vi "RasterScan.vi"() -> ()   [LabVIEW 2009]
panel:
  in  "Tab Control":T1(tab)=enum."IKI1 + NICMOS"
  in  "Aero-Me: Size":i32=5
  in  "Aero-Me: Step":dbl=50.0
  in  "Iki1: Size":i32=5
  in  "Iki1: Step":dbl=0.1
  in  "Iki2: Size":i32=5
  in  "Iki2: Step":dbl=0.1
  in  "Schnee-Me: Step":dbl=50.0
  in  "Schnee-Me: Size":i32=5
  out "Final Y":dbl
  out "Final X":dbl
  out "Start Y":dbl=53210.0
  out "Start X":dbl=24018.0
  out "Raster Scan":dbl[][](graph)
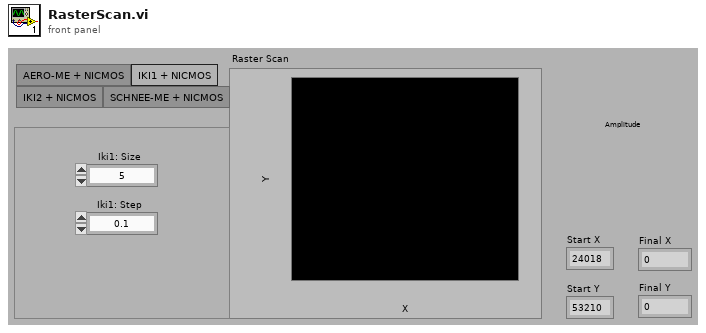
[diagram p1: front panel]
types:
  T1 = enum32{"AERO-ME + NICMOS", "IKI1 + NICMOS", "IKI2 + NICMOS", "SCHNEE-ME + NICMOS"}
  T2 = enum16{"Acquire", "GetAbsolutePosition", "AbsoluteMove", "Release"}
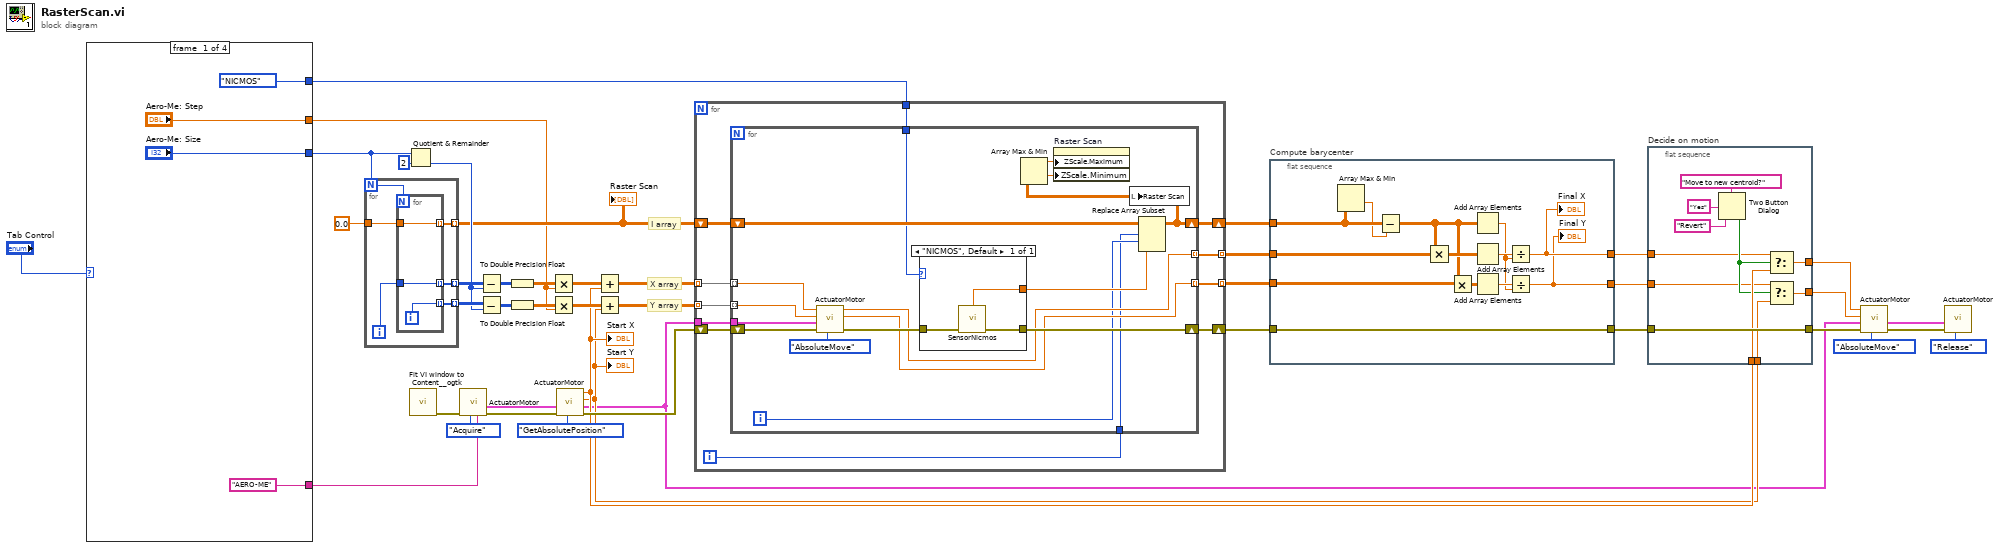
[diagram p0: block diagram]
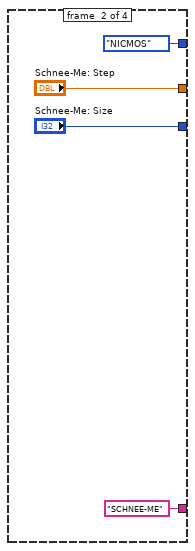
[diagram p2: hidden frame]
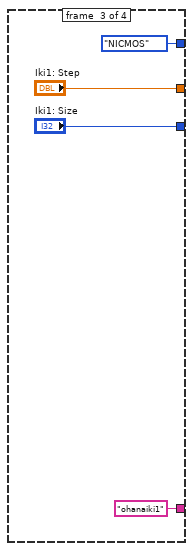
[diagram p3: hidden frame]
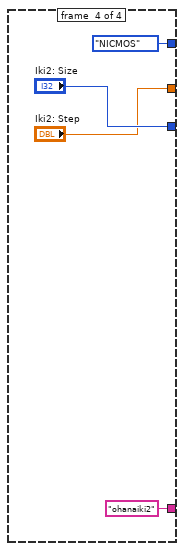
[diagram p4: hidden frame]
diagram:
  # "I array"
  # "Y array"
  # "X array"
  n1 = case shown="\"IKI2 + NICMOS\"" "Tab Control" {
    tunnel: ["Aero-Me: Size" "Schnee-Me: Size" "Iki1: Size" "Iki2: Size"] -> w40
    tunnel: ["Aero-Me: Step" "Schnee-Me: Step" "Iki1: Step" "Iki2: Step"] -> w7
    tunnel: [enum16{"NICMOS"}."NICMOS" ("Sensor") enum16{"NICMOS"}."NICMOS" ("Sensor") enum16{"NICMOS"}."NICMOS" ("Sensor") enum16{"NICMOS"}."NICMOS" ("Sensor")] -> w6
    tunnel: ["AERO-ME" ("Ring Text.Text") "SCHNEE-ME" ("Ring Text.Text") "ohanaiki1" ("Ring Text.Text") "ohanaiki2" ("Ring Text.Text")] -> w5
    frame #0 {
    }
    frame #1 {
    }
    frame #2 {
    }
    frame #3 {
    }
  }
  n2 = for {
    N: w40 -> [w61]
    tunnel: [w64] -> w42 mode=indexing
    tunnel: [w62] -> w41 mode=indexing
    tunnel: 0.0 ("element") -> [w60]
    tunnel: [w59] -> w12 mode=indexing
    i -> [w63]
    n3 = for {
      N: w61 -> [_]
      tunnel: [w67] -> w64 mode=indexing
      tunnel: w63 -> [w67]
      tunnel: [w66] -> w62 mode=indexing
      tunnel: w60 -> [w65]
      tunnel: [w65] -> w59 mode=indexing
      i -> [w66]
    }
  }
  "Raster Scan" <- w12
  n4 = Quotient & Remainder(x=w40, y=2) -> (floor(x/y)=w38:i32)  [unwired: 1 out]
  n5 = call <userlib>:"Fit VI window to Content__ogtk.vi"() -> ("error out"=w4:errorcluster)  [unwired: 6 in, 1 out]
  n6 = call "ActuatorMotor.vi"("Actuator Name"=w5, "Command"=T2."Acquire", "error in (no error)"=w4) -> ("error out"=w27:errorcluster, "RefNum out"=w3:cluster{string, "Variant":variant})  [unwired: 3 in, 2 out]
  n7 = Subtract(x=w42, y=w38) -> (x-y=w36:i32[][])
  n8 = Subtract(x=w41, y=w38) -> (x-y=w33:i32[][])
  n9 = To Double Precision Float(number=w36) -> (double precision float=w35:dbl[][])
  n10 = To Double Precision Float(number=w33) -> (double precision float=w34:dbl[][])
  n11 = Multiply(x=w35, y=w7) -> (x*y=w25:dbl[][])
  n12 = Multiply(x=w34, y=w7) -> (x*y=w23:dbl[][])
  n13 = call "ActuatorMotor.vi"("Command"=T2."GetAbsolutePosition", "error in (no error)"=w27, "RefNum"=w3) -> ("error out"=w31:errorcluster, "RefNum out"=w1:cluster{string, "Variant":variant}, "Y out"=w15:dbl, "X out"=w16:dbl)  [unwired: 3 in]
  "Start X" <- w16
  "Start Y" <- w15
  n14 = Add(x=w25, y=w16) -> (x+y=w24:dbl[][])
  n15 = Add(x=w23, y=w15) -> (x+y=w22:dbl[][])
  n16 = for {
    tunnel: w24 -> [w78] mode=indexing
    tunnel: w22 -> [w77] mode=indexing
    shift-right: [w69] -> w11
    shift-left: w12 -> [w76]
    tunnel: w6 -> [w73]
    shift-right: [w72] -> w32
    shift-left: w31 -> [w74]
    tunnel: [w71] -> w30 mode=indexing
    tunnel: [w70] -> w29 mode=indexing
    tunnel: w1 -> [w68]
    i -> [w75]
    n17 = for {
      tunnel: w78 -> [w88] mode=indexing
      tunnel: w77 -> [w87] mode=indexing
      shift-right: [w84] -> w69
      shift-left: w76 -> [w95]
      tunnel: w75 -> [w80]
      tunnel: w73 -> [w93]
      shift-right: [w90] -> w72
      shift-left: w74 -> [w92]
      tunnel: [w86] -> w71 mode=indexing
      tunnel: [w85] -> w70 mode=indexing
      tunnel: w68 -> [w79]
      i -> [w81]
      n18 = call "ActuatorMotor.vi"("Command"=T2."AbsoluteMove", "error in (no error)"=w92, "RefNum"=w79, "Y"=w87, "X"=w88) -> ("error out"=w91:errorcluster, "Y out"=w85:dbl, "X out"=w86:dbl)  [unwired: 1 in, 1 out]
      n19 = case shown="\"NICMOS\", Default" w93 {
        tunnel: [w98] -> w94
        tunnel: w91 -> [w97]
        tunnel: [w96] -> w90
        frame "NICMOS", Default {
          n20 = call "SensorNicmos.vi"("error in (no error)"=w97) -> ("error out"=w96:errorcluster, "Intensity"=w98:dbl)  [unwired: 3 in]
        }
      }
      n21 = Replace Array Subset(array=w95, new element=w94, index (row)=w80, index (col)=w81) -> (w84:dbl[][])
      n22 = Array Max & Min(array=w84) -> (max value=w83:dbl, min value=w82:dbl)  [unwired: 2 out]
      n23 = property on="Raster Scan" class="IntGraph (strict)"("ZScale.Maximum"=w83, "ZScale.Minimum"=w82) -> ()  [unwired: 2 in, 2 out]
      n24 = local write "Raster Scan"(w84) -> ()
    }
  }
  n25 = flat-sequence "Compute barycenter" {
    tunnel: w32 -> [w111]
    tunnel: [w111] -> w18
    tunnel: w30 -> [w110]
    tunnel: w29 -> [w109]
    tunnel: w11 -> [w103]
    tunnel: [w100] -> w10
    tunnel: [w99] -> w9
    frame #0 {
      n26 = Array Max & Min(array=w103) -> (min value=w101:dbl)  [unwired: 3 out]
      n27 = Subtract(x=w103, y=w101) -> (x-y=w102:dbl[][])
      n28 = Multiply(x=w102, y=w110) -> (x*y=w108:dbl[][])
      n29 = Multiply(x=w102, y=w109) -> (x*y=w107:dbl[][])
      n30 = Add Array Elements(numeric array=w102) -> (sum=w104:dbl)
      n31 = Add Array Elements(numeric array=w108) -> (sum=w106:dbl)
      n32 = Add Array Elements(numeric array=w107) -> (sum=w105:dbl)
      n33 = Divide(x=w106, y=w104) -> (x/y=w100:dbl)
      "Final X" <- w100
      n34 = Divide(x=w105, y=w104) -> (x/y=w99:dbl)
      "Final Y" <- w99
    }
  }
  n35 = flat-sequence "Decide on motion" {
    tunnel: w18 -> [w119]
    tunnel: [w119] -> w17
    tunnel: w16 -> [w115]
    tunnel: w15 -> [w116]
    tunnel: [w118] -> w14
    tunnel: [w117] -> w13
    tunnel: w10 -> [w113]
    tunnel: w9 -> [w112]
    frame #0 {
      n36 = Two Button Dialog(message="Move to new centroid?", 1:"Revert" ("F button name (\"Cancel\")"), 2:"Yes" ("T button name (\"OK\")")) -> (T button?=w114:bool)
      n37 = Select(t=w113, s=w114, f=w115) -> (s? t:f=w118:dbl)
      n38 = Select(t=w112, s=w114, f=w116) -> (s? t:f=w117:dbl)
    }
  }
  n39 = call "ActuatorMotor.vi"("Command"=T2."AbsoluteMove", "error in (no error)"=w17, "RefNum"=w1, "Y"=w13, "X"=w14) -> ("error out"=w19:errorcluster, "RefNum out"=w2:cluster{string, "Variant":variant})  [unwired: 1 in, 2 out]
  n40 = call "ActuatorMotor.vi"("Command"=T2."Release", "error in (no error)"=w19, "RefNum"=w2) -> ()  [unwired: 3 in, 4 out]
